vi "PXIe-5172Ref_Create.vi"(8 "Error In":errorcluster, 10 "PXIe-5172.lvclass":refnum<class "PXIe-5172.lvclass">, 11 "reference in":refnum<class "PXIe-5172Ref.lvclass">) -> (0 "Error Out":errorcluster, 3 "reference out":refnum<class "PXIe-5172Ref.lvclass">)   [LabVIEW 2023, in "PXIe-5172.lvlib" / "PXIe-5172Ref.lvclass"]
uses:
  PXIe-5172Ref.lvclass
  PXIe-5172.lvclass
  PXIe-5172Ref.lvclass/PXIe-5172Ref.ctl
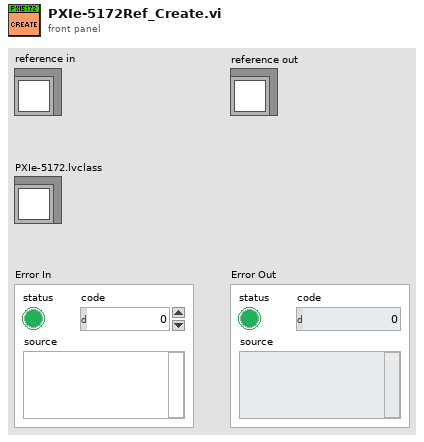
[diagram p1: front panel]
types:
  T1 = typedef "PXIe-5172.lvlib/PXIe-5172Ref.lvclass/ObjectAttributes.ctl" = cluster{"PXIe-5172.lvclass":refnum<class "PXIe-5172.lvclass">}
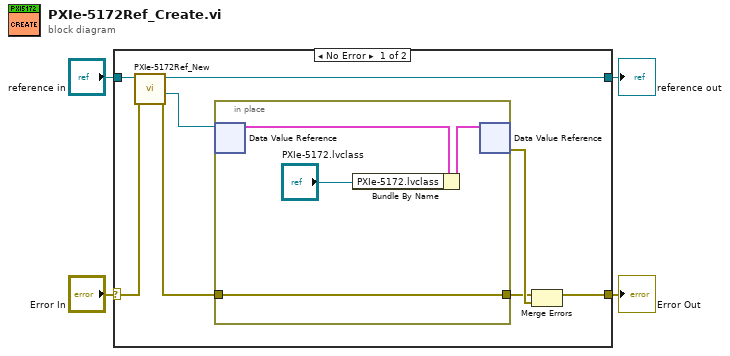
[diagram p0: block diagram]
diagram:
  n1 = case shown="No Error" "Error In" {
    selector: "Error In" -> [w11 w18]
    tunnel: [w5 w18] -> w3
    tunnel: "reference in" -> [w12 w17]
    tunnel: [w10 w17] -> w1
    frame No Error {
      n2 = call "PXIe-5172Ref_New.vi"("Error In"=w11, "reference in"=w12) -> ("Error Out"=w7:errorcluster, "DVRRefOut"=w8:refnum<data-value>, "reference out"=w10:refnum<class "PXIe-5172Ref.lvclass">)  [unwired: 6 in, 1 out]
      n3 = in-place {
        in-place-border: w7 -> [w14]
        in-place-border: [w14] -> w6
        n4 = in-place-dvr #1(w8) -> (w15:T1)  [unwired: 1 out]
        n5 = Bundle By Name(cluster=w15, "PXIe-5172.lvclass"="PXIe-5172.lvclass") -> (w16:T1)
        n6 = in-place-dvr #1(w16) -> (w9:errorcluster)  [unwired: 1 out]
      }
      n7 = Merge Errors(w6, w9) -> (w5:errorcluster)
    }
    frame Error {
      # "VI-TechBaseTemplate_Simple_4x4x4"
    }
  }
  "Error Out" <- w3
  "reference out" <- w1
